vi "Read Magnetometer I2C.vi"(8 "error in (no error)":errorcluster, 11 "LSM9DS1 IMU in":refnum<class "LSM9DS1 IMU.lvclass">) -> (0 "error out":errorcluster, 2 "LINX I2C":refnum<class "LINX I2C.lvclass">, 3 "LSM9DS1 IMU out":refnum<class "LSM9DS1 IMU.lvclass">)   [LabVIEW 2020, in "LSM9DS1 IMU.lvclass"]
uses:
  LSM9DS1 IMU.lvclass
  LINX I2C/LINX I2C.lvclass
  LSM9DS1 IMU.lvclass/LSM9DS1 IMU.ctl
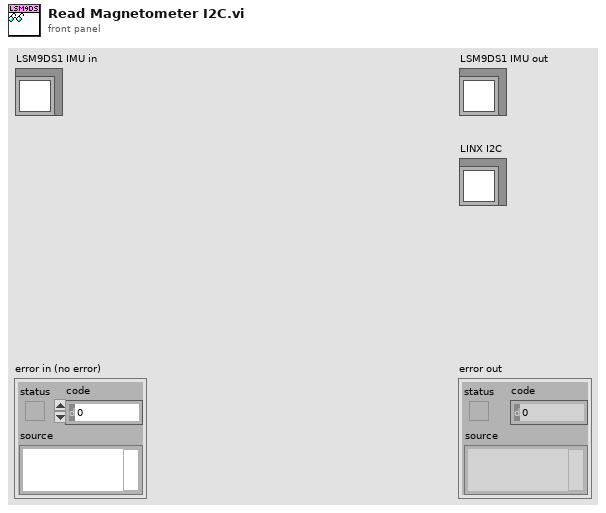
[diagram p1: front panel]
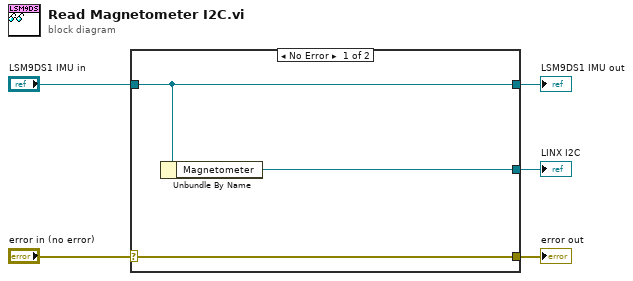
[diagram p0: block diagram]
diagram:
  n1 = case shown="No Error" "error in (no error)" {
    selector: "error in (no error)" -> [w8 w9]
    tunnel: [w8 w9] -> w4
    tunnel: [w7 w10] -> w2
    tunnel: "LSM9DS1 IMU in" -> [w7 w10]
    tunnel: [w6 _] -> w1
    frame No Error {
      n2 = Unbundle By Name(w7) -> ("Magnetometer"=w6:refnum<class "LINX I2C.lvclass">)
    }
    frame Error {
    }
  }
  "error out" <- w4
  "LSM9DS1 IMU out" <- w2
  "LINX I2C" <- w1
